vi "flash.vi"   [LabVIEW 2017]
uses:
  globalUtilities.vi
types:
  T1 = cluster{"button info":cluster{"button 1":bool, "button 2":bool, "button 3":bool, "button 4":bool, "button 5":bool, "button 6":bool, "button 7":bool, "button 8":bool, "button 9":bool, "button 10":bool, "button 11":bool, "button 12":bool, "button 13":bool, "button 14":bool, "button 15":bool, "button 16":bool, "button 17":bool, "button 18":bool, "button 19":bool, "button 20":bool, "button 21":bool, "button 22":bool, "button 23":bool, "button 24":bool, "button 25":bool, "button 26":bool, "button 27":bool, "button 28":bool, "button 29":bool, "button 30":bool, "button 31":bool, "button 32":bool}, "direction info":cluster{"pov 1":i32, "pov 2":i32, "pov 3":i32, "pov 4":i32}, "axis info":cluster{"X axis":i32, "Y axis":i32, "Z axis":i32, "X axis rotation":i32, "Y axis rotation":i32, "Z axis rotation":i32, "U axis":i32, "V axis":i32}}
  T2 = cluster{"button 1":bool, "button 2":bool, "button 3":bool, "button 4":bool, "button 5":bool, "button 6":bool, "button 7":bool, "button 8":bool, "button 9":bool, "button 10":bool, "button 11":bool, "button 12":bool, "button 13":bool, "button 14":bool, "button 15":bool, "button 16":bool, "button 17":bool, "button 18":bool, "button 19":bool, "button 20":bool, "button 21":bool, "button 22":bool, "button 23":bool, "button 24":bool, "button 25":bool, "button 26":bool, "button 27":bool, "button 28":bool, "button 29":bool, "button 30":bool, "button 31":bool, "button 32":bool}
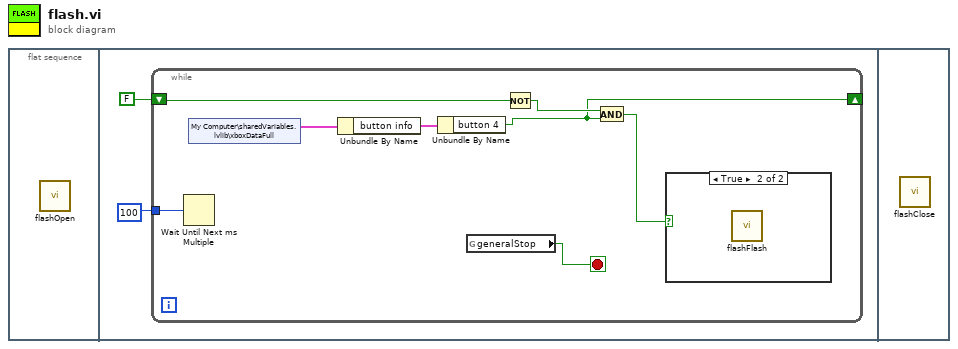
[diagram p0: block diagram]
diagram:
  n1 = flat-sequence {
    frame #0 {
      n2 = call "flashOpen.vi"() -> ()  [unwired: 12 in]
    }
    frame #1 {
      n3 = while {
        tunnel: 100 -> [w10]
        shift-right: [w3] -> _
        shift-left: FALSE -> [w6]
        stop <- w9 stop-if-true
        n4 = Wait Until Next ms Multiple(millisecond multiple=w10) -> ()  [unwired: 1 out]
        n5 = shared-variable "My Computer\\sharedVariables.lvlib\\xboxDataFull"() -> (w8:T1)  [unwired: 1 in, 1 out]
        n6 = Unbundle By Name(w8) -> ("button info"=w7:T2)
        n7 = Unbundle By Name(w7) -> ("button 4"=w3:bool)
        n8 = global read "globalUtilities.vi" "generalStop"() -> (w9:bool)
        n9 = Not(x=w6) -> (.not. x?=w5:bool)
        n10 = And(x=w5, y=w3) -> (x .and. y?=w4:bool)
        n11 = case shown="True" w4 {
          frame False {
          }
          frame True {
            n12 = call "flashFlash.vi"() -> ()  [unwired: 12 in]
          }
        }
      }
    }
    frame #2 {
      n13 = call "flashClose.vi"() -> ()  [unwired: 12 in]
    }
  }
